vi "Creator.vi"(7 "jettl in":refnum<class "jettl.lvclass">, 8 "Priority?":bool, 9 "Msg Strategy":refnum<class "Msg Strategy.lvclass">, 10 "Addresses DVR":refnum<data-value>) -> (5 "jettl out":refnum<class "jettl.lvclass">)   [LabVIEW 2021, in "jettl.lvlib" / "Addresses.lvlib"]
uses:
  Addresses.lvlib
  jettl/jettl.lvclass
  Msg Type Strategy/Msg Type Strategy/Msg Type Strategy.lvclass
  Msg Strategy/Msg Strategy.lvclass
  Addresses/Addresses.lvclass
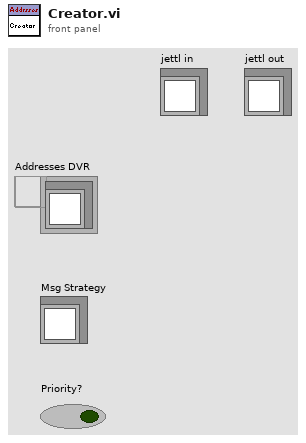
[diagram p1: front panel]
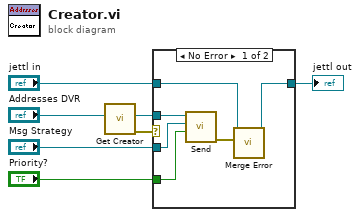
[diagram p0: block diagram]
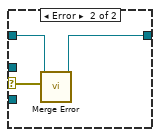
[diagram p2: hidden frame]
diagram:
  n1 = call "Get Creator.vi"("Addresses DVR"="Addresses DVR") -> ("error out"=w1:errorcluster, "Creator"=w5:refnum<class "Msg Type Strategy.lvclass">)  [unwired: 9 in]
  n2 = case shown="No Error" w1 {
    selector: w1 -> [_ w14]
    tunnel: "Msg Strategy" -> [w9 _]
    tunnel: "Priority?" -> [w8 _]
    tunnel: w5 -> [w10 _]
    tunnel: "jettl in" -> [w12 w16]
    tunnel: [w11 w15] -> w2
    frame No Error {
      n3 = call-dynamic "Send.vi"("Priority?"=w8, "Msg Strategy"=w9, "Msg Type Strategy in"=w10) -> ("error out"=w13:errorcluster)  [unwired: 8 in]
      n4 = call-dynamic "Merge Error.vi"("Error"=w13, "Merge Error in"=w12) -> ("Merge Error out"=w11:refnum<class "jettl.lvclass">)  [unwired: 9 in]
    }
    frame Error {
      n5 = call-dynamic "Merge Error.vi"("Error"=w14, "Merge Error in"=w16) -> ("Merge Error out"=w15:refnum<class "jettl.lvclass">)  [unwired: 9 in]
    }
  }
  "jettl out" <- w2
